vi "Is Sensor Healthy.vi"(11 "Sensor Value":u32) -> (3 "Healthy":bool)   [LabVIEW 2014]
uses:
  Controls/Sensor Healthy.ctl
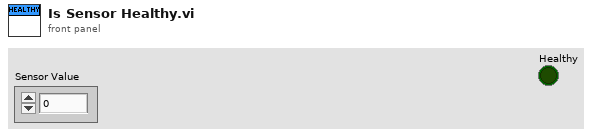
[diagram p1: front panel]
types:
  T1 = typedef "Sensor Healthy.ctl" = u32
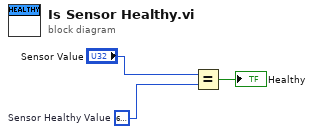
[diagram p0: block diagram]
diagram:
  w2 = T1 6618880  # Sensor Healthy Value
  n1 = Equal?(x="Sensor Value", y=w2) -> (x = y?=→"Healthy":bool)
